vi "SINGLESYRINGEPUMP.vi"() -> ()   [LabVIEW 2020]
panel:
  in  "repeat":i32
  in  "pause 1 (ms)":u32=10000
  in  "VISA resource name 2":refnum<visa-resource-name>
  in  "error in (no error) 1":errorcluster
  out "VISA resource name 1":refnum<visa-resource-name>
  out "error out 1":errorcluster
  out "read buffer 1":string
  out "return count 1":u32
  out "VISA resource name out 1":refnum<visa-resource-name>
  out "output string 1":string
  in  "multi-line string 1":string
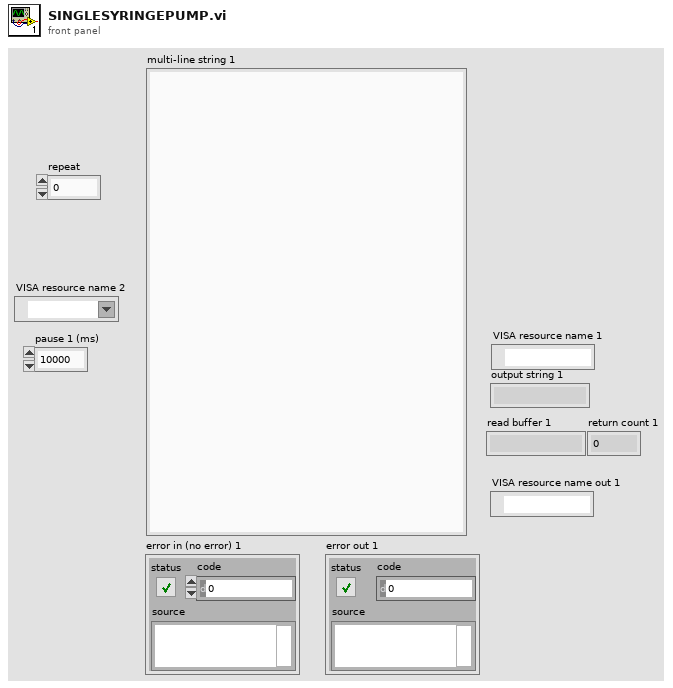
[diagram p1: front panel]
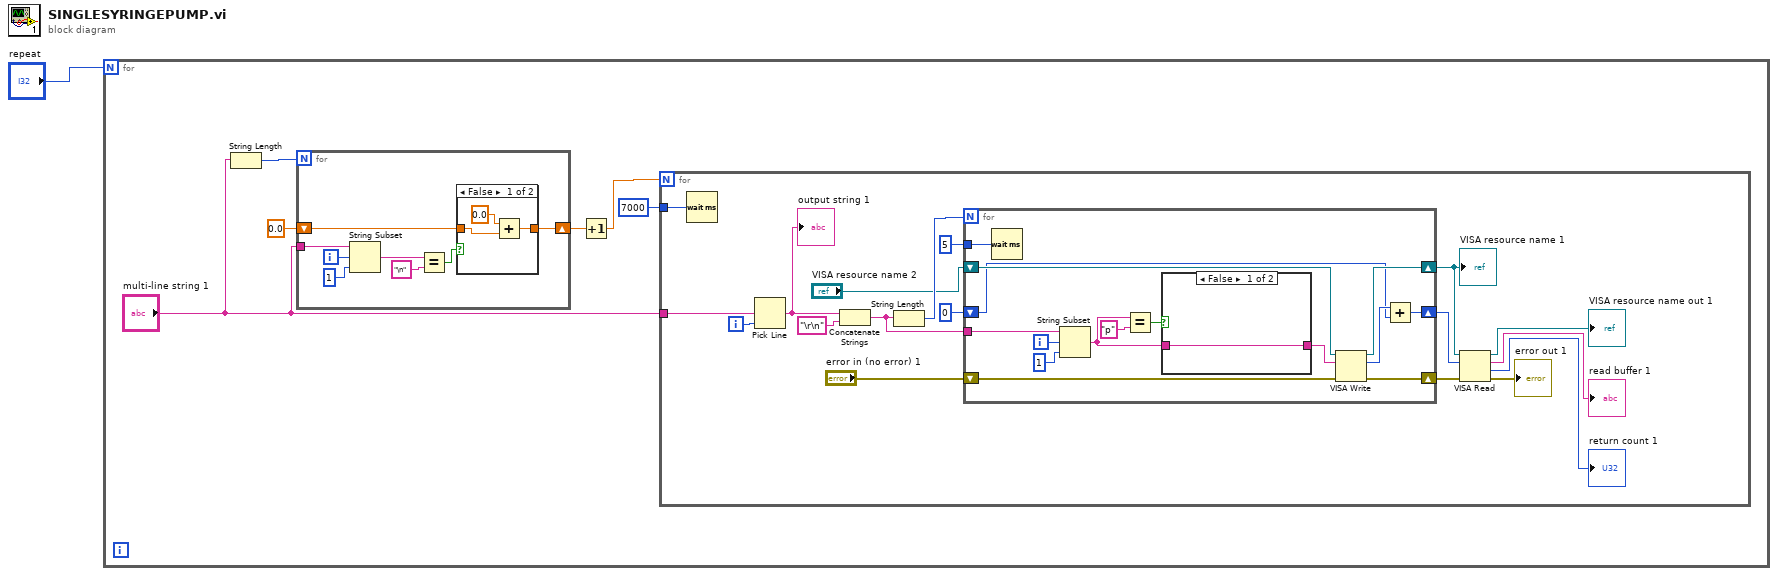
[diagram p0: block diagram]
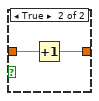
[diagram p2: hidden frame]
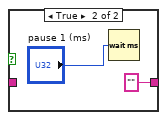
[diagram p3: hidden frame]
diagram:
  n1 = for {
    N: "repeat" -> [_]
    n2 = String Length(string="multi-line string 1") -> (length=w5:i32)
    n3 = for {
      N: w5 -> [_]
      tunnel: "multi-line string 1" -> [w13]
      shift-right: [w8] -> w4
      shift-left: 0.0 ("x") -> [w9]
      i -> [w14]
      n4 = String Subset(string=w13, offset (0)=w14, length (rest)=1 ("length (rest)")) -> (substring=w12:string)
      n5 = Equal?(x=w12, y="\n") -> (x = y?=w10:bool)
      n6 = case shown="False" w10 {
        tunnel: w9 -> [w17 w20]
        tunnel: [w16 w19] -> w8
        frame False {
          n7 = Add(x=0.0 ("x+y"), y=w17) -> (x+y=w16:dbl)
        }
        frame True {
          n8 = Increment(x=w20) -> (x+1=w19:dbl)
        }
      }
    }
    n9 = Increment(x=w4) -> (x+1=w3:dbl)
    n10 = for {
      N: w3 -> [_]
      tunnel: "multi-line string 1" -> [w27]
      tunnel: u32 7000 ("milliseconds to wait") -> [w21]
      i -> [w26]
      n11 = Wait (ms)(milliseconds to wait=w21) -> ()  [unwired: 1 out]
      n12 = Pick Line(multi-line string=w27, line index=w26) -> (output string=w23:string)  [unwired: 1 in]
      "output string 1" <- w23
      n13 = Concatenate Strings(w23, "\r\n" ("string")) -> (w24:string)
      n14 = String Length(string=w24) -> (length=w38:i32)
      n15 = for {
        N: w38 -> [_]
        tunnel: w24 -> [w53]
        tunnel: u32 5 ("milliseconds to wait") -> [w49]
        shift-right: [w47] -> w28
        shift-left: "VISA resource name 2" -> [w51]
        shift-right: [w46] -> w32
        shift-left: "error in (no error) 1" -> [w50]
        shift-right: [w44] -> w33
        shift-left: u32 0 ("y") -> [w45]
        i -> [w52]
        n16 = Wait (ms)(milliseconds to wait=w49) -> ()  [unwired: 1 out]
        n17 = String Subset(string=w53, offset (0)=w52, length (rest)=1 ("length (rest)")) -> (substring=w39:string)
        n18 = Equal?(x=w39, y="p") -> (x = y?=w42:bool)
        n19 = case shown="False" w42 {
          tunnel: [w54 ""] -> w40
          tunnel: w39 -> [w54 _]
          frame False {
          }
          frame True {
            n20 = Wait (ms)(milliseconds to wait="pause 1 (ms)") -> ()  [unwired: 1 out]
          }
        }
        n21 = VISA Write(VISA resource name=w51, write buffer=w40, error in (no error)=w50) -> (VISA resource name out=w47:refnum<visa-resource-name>, return count=w48:u32, error out=w46:errorcluster)
        n22 = Add(x=w48, y=w45) -> (x+y=w44:u32)
      }
      "VISA resource name 1" <- w28
      n23 = VISA Read(VISA resource name=w28, byte count=w33, error in (no error)=w32) -> (VISA resource name out=→"VISA resource name out 1":refnum<visa-resource-name>, read buffer=→"read buffer 1":string, return count=→"return count 1":u32, error out=→"error out 1":errorcluster)
    }
  }
